vi "PixelatedDetectorP1New.vi"() -> ()   [LabVIEW 2018]
panel:
  out "Intensity Graph":dbl[][](graph)
  in  "velocity":dbl
  in  "bField":dbl
  out "XY Graph":cluster{dbl[], dbl[]}(graph)
  in  "height":dbl
  in  "eField":dbl
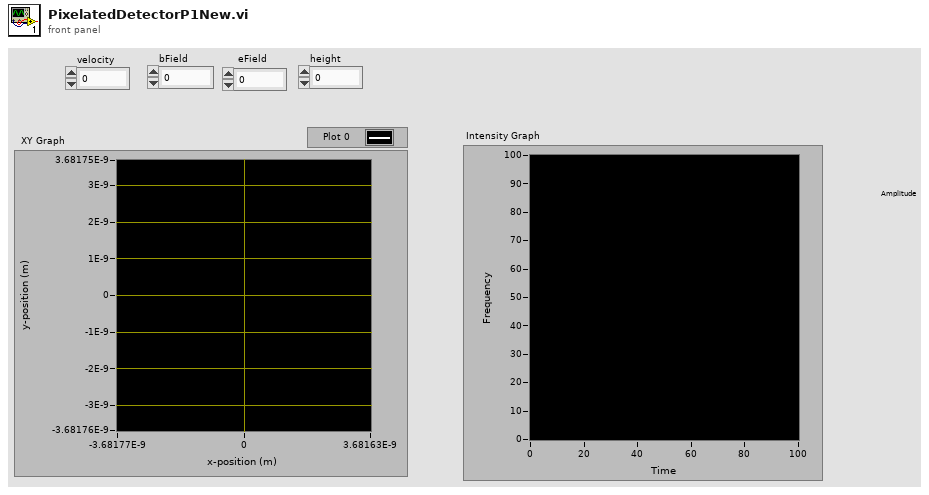
[diagram p1: front panel]
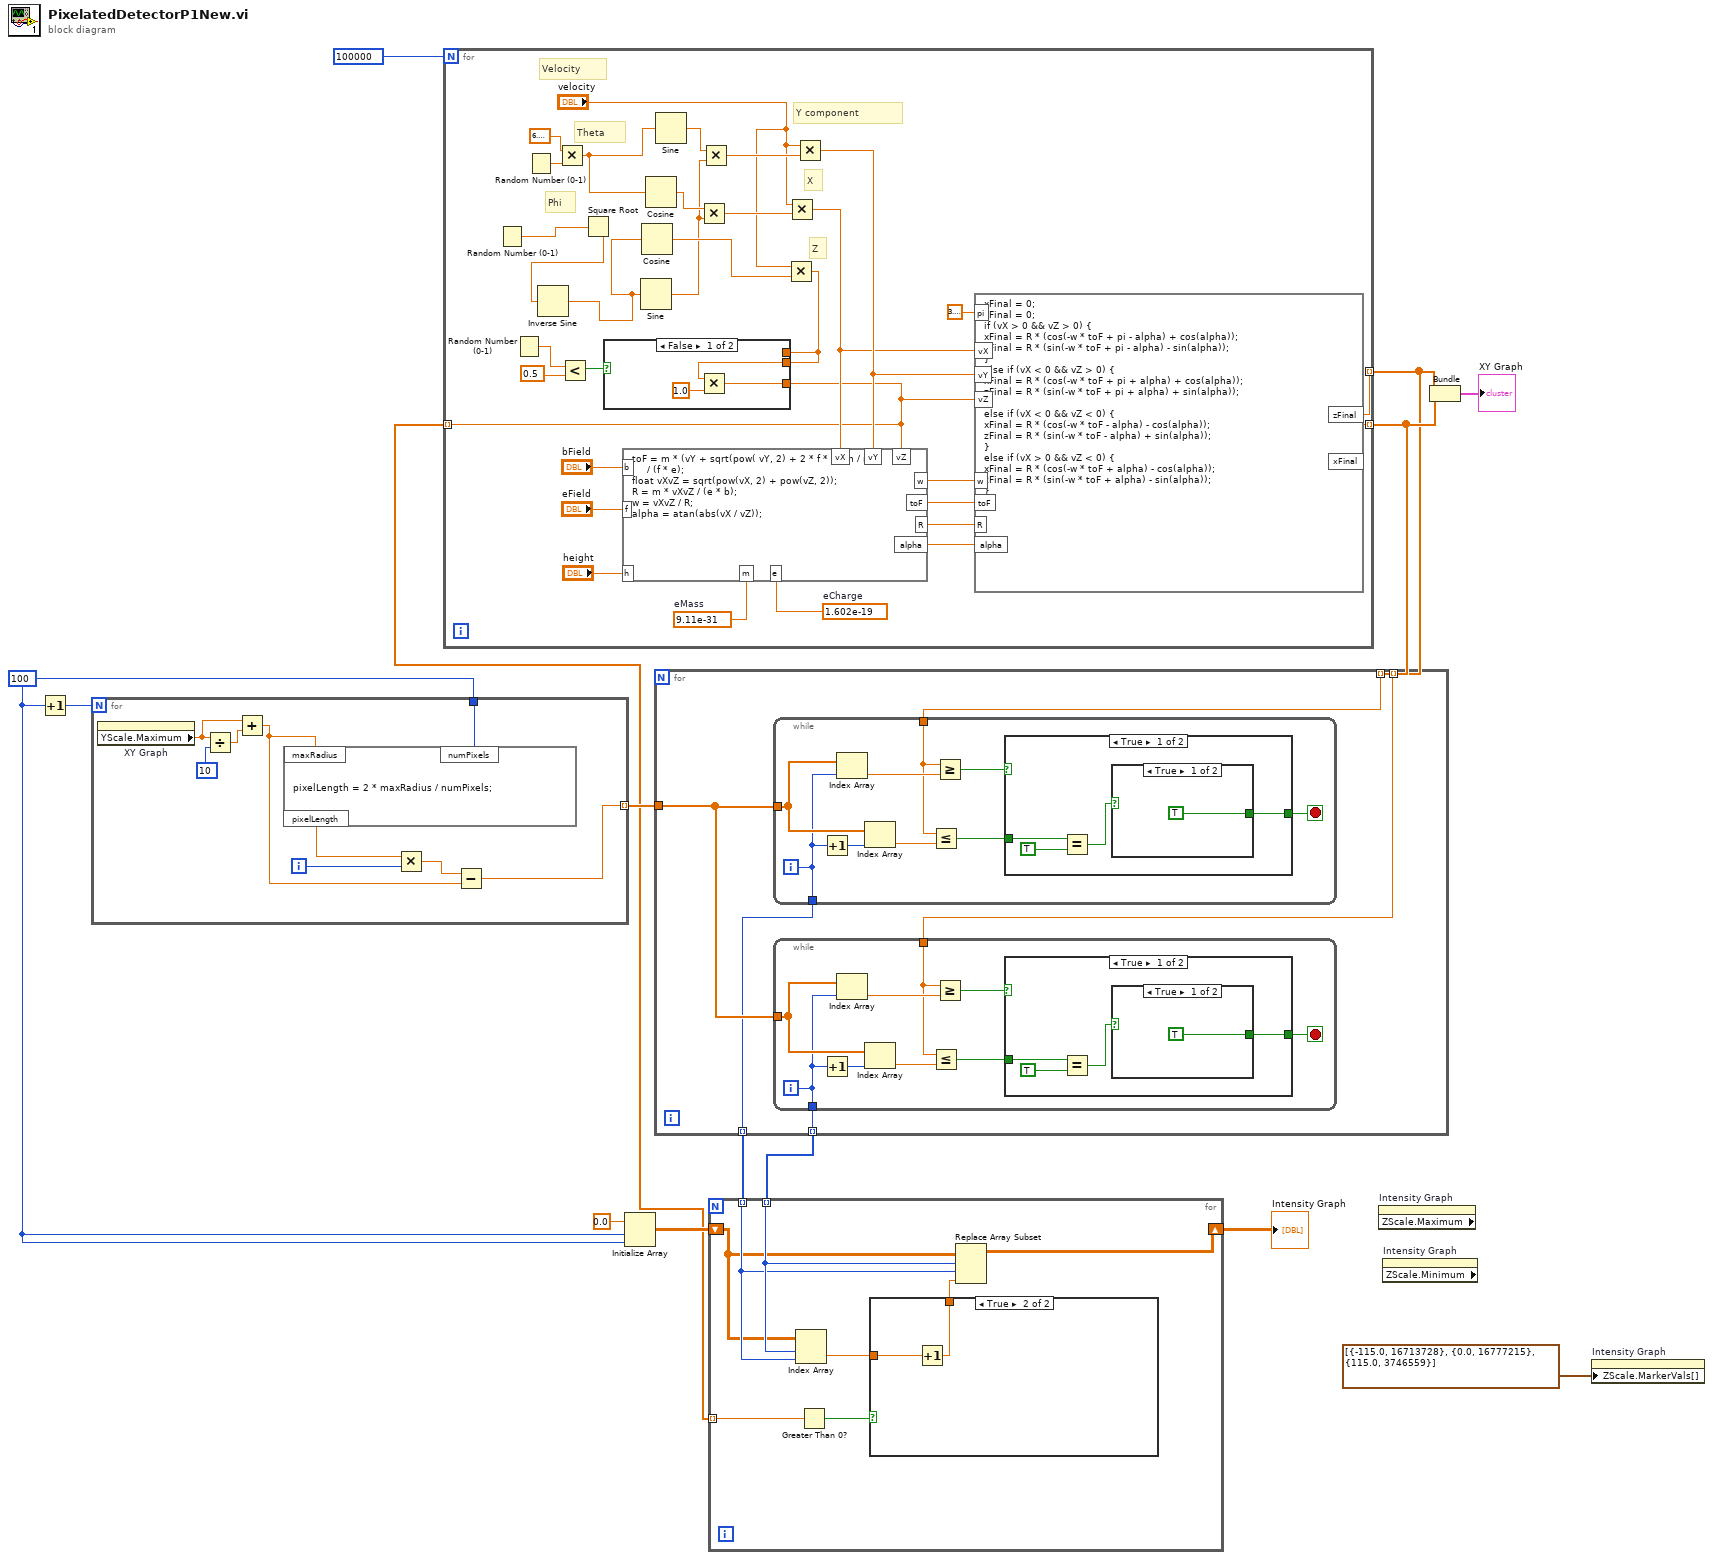
[diagram p0: block diagram]
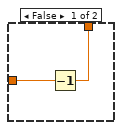
[diagram p2: hidden frame]
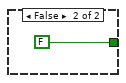
[diagram p3: hidden frame]
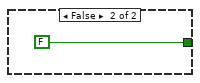
[diagram p4: hidden frame]
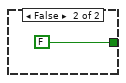
[diagram p5: hidden frame]
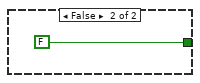
[diagram p6: hidden frame]
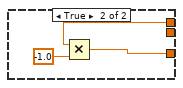
[diagram p7: hidden frame]
diagram:
  w7 = 100
  n1 = Increment(x=w7) -> (x+1=w13:i32)
  n2 = for {
    N: w13 -> [_]
    tunnel: [w19] -> w8 mode=indexing
    tunnel: w7 -> [w23]
    i -> [w22]
    n3 = property on="XY Graph" class="XYGraph (strict)"() -> ("YScale.Maximum"=w16:dbl)  [unwired: 2 in, 2 out]
    n4 = Divide(x=w16, y=10) -> (x/y=w17:dbl)
    n5 = Add(x=w16, y=w17) -> (x+y=w15:dbl)
    n6 = formula code="pixelLength = 2 * maxRadius / numPixels;"("numPixels"=w23, "maxRadius"=w15) -> ("pixelLength"=w21:dbl)
    n7 = Multiply(x=w21, y=w22) -> (x*y=w20:dbl)
    n8 = Subtract(x=w20, y=w15) -> (x-y=w19:dbl)
  }
  n9 = for {
    N: 100000 -> [_]
    tunnel: [w51] -> w11 mode=indexing
    tunnel: [w50] -> w12 mode=indexing
    tunnel: [w24] -> w3 mode=indexing
    w25 = 9.11e-31  # eMass
    w26 = 1.602e-19  # eCharge
    # "Phi"
    # "Theta"
    # "Z"
    # "X"
    # "Y component"
    # "Velocity"
    n10 = Random Number (0-1)() -> (number: 0 to 1=w31:dbl)
    n11 = Random Number (0-1)() -> (number: 0 to 1=w37:dbl)
    n12 = Random Number (0-1)() -> (number: 0 to 1=w46:dbl)
    n13 = Multiply(x=6.283185307179586, y=w46) -> (x*y=w44:dbl)
    n14 = Less?(x=w37, y=0.5) -> (x < y?=w35:bool)
    n15 = Square Root(x=w31) -> (sqrt(x)=w32:dbl)
    n16 = Inverse Sine(1:w32) -> (0:w33:dbl)
    n17 = Sine(x=w33) -> (sin(x)=w39:dbl)
    n18 = Cosine(x=w33) -> (cos(x)=w43:dbl)
    n19 = Cosine(x=w44) -> (cos(x)=w40:dbl)
    n20 = Sine(x=w44) -> (sin(x)=w42:dbl)
    n21 = Multiply(x=w40, y=w39) -> (x*y=w38:dbl)
    n22 = Multiply(x=w42, y=w39) -> (x*y=w41:dbl)
    n23 = Multiply(x="velocity", y=w43) -> (x*y=w34:dbl)
    n24 = case shown="False" w35 {
      tunnel: [w57 w61] -> w24
      tunnel: w34 -> [w56 _]
      tunnel: w34 -> [_ w59]
      frame False {
        n25 = Multiply(x=w56, y=1.0) -> (x*y=w57:dbl)
      }
      frame True {
        n26 = Multiply(x=w59, y=-1.0) -> (x*y=w61:dbl)
      }
    }
    n27 = Multiply(x="velocity", y=w38) -> (x*y=w29:dbl)
    n28 = Multiply(x="velocity", y=w41) -> (x*y=w30:dbl)
    n29 = formula code="toF = m * (vY + sqrt(pow( vY, 2) + 2 * f * e * h / m))\n     / (f * e);\nfloat vXvZ = sqrt(pow(vX, 2) + pow(vZ, 2));\nR = m * vXvZ / (e * b);\nw = vXvZ / R;\nalpha = atan(abs(vX / vZ));"("f"="eField", "h"="height", "vY"=w30, "m"=w25, "e"=w26, "vX"=w29, "vZ"=w24, "b"="bField") -> ("toF"=w54:dbl, "w"=w53:dbl, "R"=w48:dbl, "alpha"=w52:dbl)
    n30 = formula code="xFinal = 0;\nzFinal = 0;\nif (vX > 0 && vZ > 0) {\nxFinal = R * (cos(-w * toF + pi - alpha) + cos(alpha));\nzFinal = R * (sin(-w * toF + pi - alpha) - sin(alpha));\n}\nelse if (vX < 0 && vZ > 0) {\nxFinal = R * (cos(-w * toF + pi + alpha) + cos(alpha));\nzFinal = R * (sin(-w * toF + pi + alpha) + sin(alpha));\n}\nelse if (vX < 0 && vZ < 0) {\nxFinal = R * (cos(-w * toF - alpha) - cos(alpha));\nzFinal = R * (sin(-w * toF - alpha) + sin(alpha));\n}\nelse if (vX > 0 && vZ < 0) {\nxFinal = R * (cos(-w * toF + alpha) - cos(alpha));\nzFinal = R * (sin(-w * toF + alpha) - sin(alpha));\n}"("vY"=w30, "toF"=w54, "vX"=w29, "vZ"=w24, "w"=w53, "R"=w48, "alpha"=w52, "pi"=3.141592653589793) -> ("zFinal"=w51:dbl, "xFinal"=w50:dbl)
  }
  n31 = Initialize Array(0.0, w7, w7) -> (w6:dbl[][])
  n32 = for {
    tunnel: w12 -> [w66] mode=indexing
    tunnel: w11 -> [w65] mode=indexing
    tunnel: w8 -> [w64]
    tunnel: [w63] -> w5 mode=indexing
    tunnel: [w62] -> w4 mode=indexing
    n33 = while {
      tunnel: w64 -> [w91]
      tunnel: w66 -> [w88]
      tunnel: [w85] -> w63
      i -> [w85]
      stop <- w84 stop-if-true
      n34 = Increment(x=w85) -> (x+1=w90:i32)
      n35 = Index Array(array=w91, index=w85) -> (element=w89:dbl)
      n36 = Index Array(array=w91, index=w90) -> (element=w87:dbl)
      n37 = Less Or Equal?(x=w88, y=w87) -> (x <= y?=w86:bool)
      n38 = Greater Or Equal?(x=w88, y=w89) -> (x >= y?=w83:bool)
      n39 = case shown="True" w83 {
        tunnel: w86 -> [w94 _]
        tunnel: [w92 FALSE] -> w84
        frame True {
          n40 = Equal?(x=w94, y=TRUE) -> (x = y?=w93:bool)
          n41 = case shown="True" w93 {
            tunnel: [TRUE FALSE] -> w92
            frame True {
            }
            frame False {
            }
          }
        }
        frame False {
        }
      }
    }
    n42 = while {
      tunnel: w64 -> [w75]
      tunnel: w65 -> [w72]
      tunnel: [w69] -> w62
      i -> [w69]
      stop <- w68 stop-if-true
      n43 = Increment(x=w69) -> (x+1=w74:i32)
      n44 = Index Array(array=w75, index=w69) -> (element=w73:dbl)
      n45 = Index Array(array=w75, index=w74) -> (element=w71:dbl)
      n46 = Less Or Equal?(x=w72, y=w71) -> (x <= y?=w70:bool)
      n47 = Greater Or Equal?(x=w72, y=w73) -> (x >= y?=w67:bool)
      n48 = case shown="True" w67 {
        tunnel: w70 -> [w78 _]
        tunnel: [w76 FALSE] -> w68
        frame True {
          n49 = Equal?(x=w78, y=TRUE) -> (x = y?=w77:bool)
          n50 = case shown="True" w77 {
            tunnel: [TRUE FALSE] -> w76
            frame True {
            }
            frame False {
            }
          }
        }
        frame False {
        }
      }
    }
  }
  n51 = for {
    tunnel: w4 -> [w106] mode=indexing
    tunnel: w5 -> [w105] mode=indexing
    shift-right: [w101] -> w2
    shift-left: w6 -> [w102]
    tunnel: w3 -> [w100] mode=indexing
    n52 = Index Array(array=w102, index (row)=w106, index (col)=w105) -> (element=w103:dbl)
    n53 = Greater Than 0?(x=w100) -> (x > 0?=w99:bool)
    n54 = case shown="True" w99 {
      tunnel: [w107 w110] -> w104
      tunnel: w103 -> [w108 w109]
      frame False {
        n55 = Decrement(x=w108) -> (x-1=w107:dbl)
      }
      frame True {
        n56 = Increment(x=w109) -> (x+1=w110:dbl)
      }
    }
    n57 = Replace Array Subset(array=w102, new element=w104, index (row)=w106, index (col)=w105) -> (w101:dbl[][])
  }
  "Intensity Graph" <- w2
  n58 = property on="Intensity Graph" class="IntGraph (strict)" props=["ZScale", "Maximum"]() -> ()  [unwired: 2 in, 3 out]
  n59 = property on="Intensity Graph" class="IntGraph (strict)" props=["ZScale", "Minimum"]() -> ()  [unwired: 2 in, 3 out]
  n60 = Bundle(w11, w12) -> (→"XY Graph":cluster{dbl[], dbl[]})  [unwired: 1 in]
  n61 = property on="Intensity Graph" class="IntGraph (strict)"("ZScale.MarkerVals[]"=cluster{dbl, u32}[] [{-115.0, 16713728}, {0.0, 16777215}, {115.0, 3746559}] ("Z Scale.Marker Values[]")) -> ()  [unwired: 2 in, 2 out]
